vi "Sprinkler.vi"() -> ()   [LabVIEW 2020]
uses:
  Controls/ZoneSetupArray.ctl
  Controls/SprinklerStates.ctl
  <vilib>/Utility/file.llb/Read Delimited Spreadsheet (string).vi
panel:
  in  "Zone Setup Array":T1
  out "Controller Status":string
  out "Zone Indicators":T2
  in  "Water Pressure Sensor (%)":u32(slide) scale=0.0..100.0
  in  "Rain Sensor":bool
  in  "Run Selector":bool
  in  "Setup":bool
  in  "Start":bool
  in  "stop":bool
  # "Controls"
  # "Simulation Controls"
  # "Rain"
  # "No Rain"
  # "Continuous"
  # "Single"
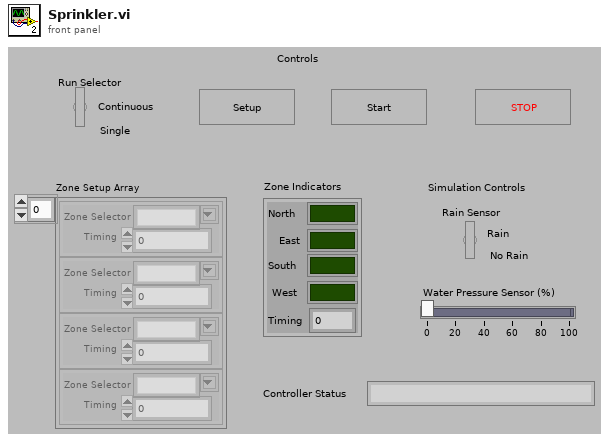
[diagram p1: front panel]
types:
  T1 = typedef "ZoneSetupArray.ctl" = cluster{"Zone Selector":string, "Timing":dbl}[]
  T2 = cluster{"North":bool, "East":bool, "South":bool, "West":bool, "Timing":u32}
  T3 = typedef "SprinklerStates.ctl" = cluster{enum16{"Default", "Init", "Setup", "Start", "Stop"}, variant}
  T4 = enum8{"Enabled", "Disabled", "Disabled and Grayed Out"}
  T5 = enum16{"Default", "Init", "Setup", "Start", "Stop"}
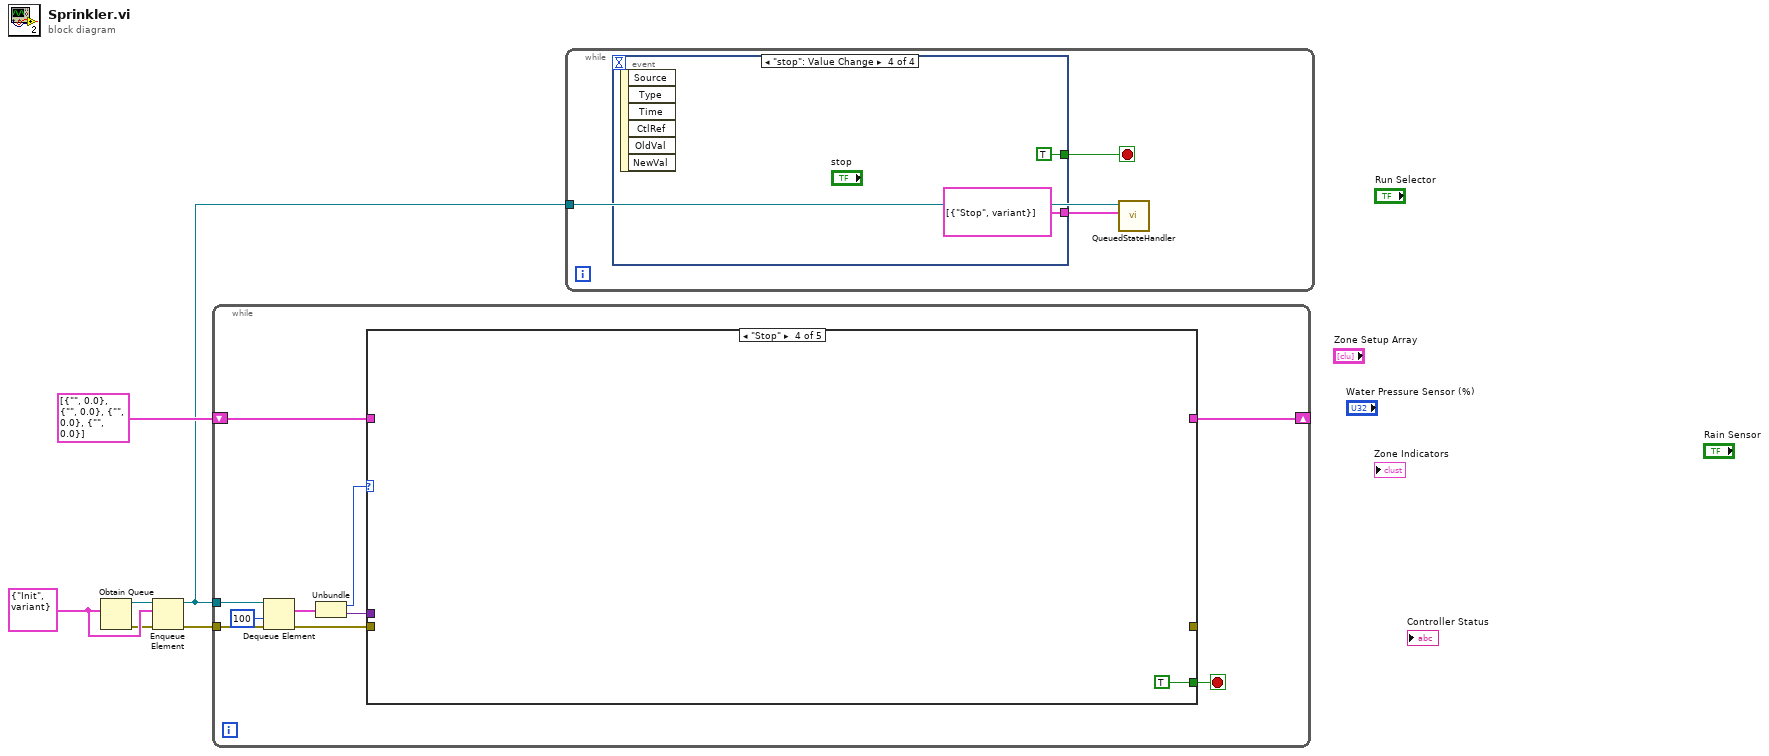
[diagram p0: block diagram]
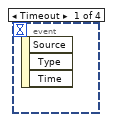
[diagram p2: hidden frame]
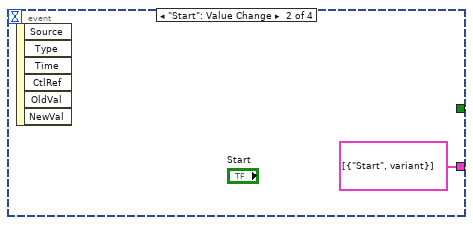
[diagram p3: hidden frame]
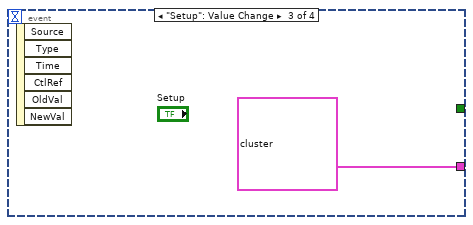
[diagram p4: hidden frame]
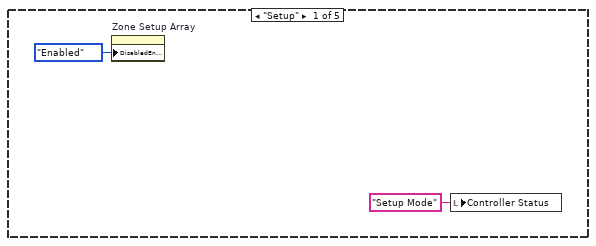
[diagram p5: hidden frame]
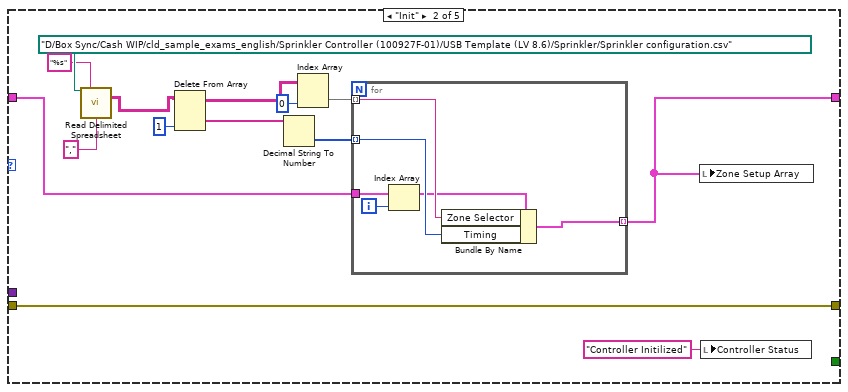
[diagram p6: hidden frame]
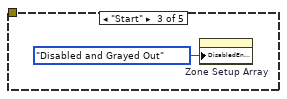
[diagram p7: hidden frame]
diagram:
  w5 = T3 {enum."Init", variant}
  n1 = Obtain Queue(element data type=w5) -> (queue out=w6:refnum<queue>, error out=w4:errorcluster)  [unwired: 4 in, 1 out]
  n2 = Enqueue Element(queue=w6, element=w5, error in (no error)=w4) -> (queue out=w1:refnum<queue>, error out=w3:errorcluster)  [unwired: 1 in, 1 out]
  n3 = while {
    tunnel: w1 -> [w16]
    tunnel: w3 -> [w15]
    shift-right: [w9] -> _
    shift-left: T1 [{"Zone Selector"="", "Timing"=0.0}, {"Zone Selector"="", "Timing"=0.0}, {"Zone Selector"="", "Timing"=0.0}, {"Zone Selector"="", "Timing"=0.0}] ("Zone Setup Array") -> [w10]
    stop <- w7 stop-if-true
    n4 = Dequeue Element(queue=w16, timeout in ms (-1)=100, error in (no error)=w15) -> (element=w13:T3, error out=w8:errorcluster)  [unwired: 2 out]
    n5 = Unbundle(w13) -> (w12:T5, w11:variant)
    n6 = case shown="\"Stop\"" w12 {
      tunnel: w11 -> [_ _ _ _ _]
      tunnel: w10 -> [_ w22 _ _ _]
      tunnel: [_ w20 _ _ _] -> w9
      tunnel: w8 -> [_ w21 _ _ _]
      tunnel: [_ w21 _ _ _] -> _
      tunnel: [_ _ _ TRUE _] -> w7
      frame "Setup" {
        n7 = property on="Zone Setup Array" class="Arr (strict)"("DisabledEnum"=T4."Enabled" ("Disabled")) -> ()  [unwired: 2 in, 2 out]
        n8 = local write "Controller Status"("Setup Mode" ("Controller Status")) -> ()
      }
      frame "Init" {
        n9 = call-poly <vilib>:"Read Delimited Spreadsheet.vi"("file path (dialog if empty)"=path "D:/Box Sync/Cash WIP/cld_sample_exams_english/Sprinkler Controller (100927F-01)/USB Template (LV 8.6)/Sprinkler/Sprinkler configuration.csv", "format (%s)"="%s" ("format (%d)"), "delimiter (\\t)"="," ("delimiter (\\t)")) -> ("all rows"=w27:string[][])  [unwired: 7 in, 5 out]
        n10 = Delete From Array(array=w27, index (col)=1 ("disabled index (col)")) -> (deleted portion=w29:string[], array with subset deleted=w25:string[][])  [unwired: 2 in]
        n11 = Decimal String To Number(string=w29) -> (number=w26:i32[])  [unwired: 2 in, 1 out]
        n12 = Index Array(array=w25, index (col)=0 ("disabled index (col)")) -> (element=w24:string[])  [unwired: 1 in]
        n13 = for {
          tunnel: w22 -> [w37]
          tunnel: [w38] -> w20 mode=indexing
          tunnel: w26 -> [w36] mode=indexing
          tunnel: w24 -> [w35] mode=indexing
          i -> [w33]
          n14 = Index Array(array=w37, index=w33) -> (element=w34:cluster{"Zone Selector":string, "Timing":dbl})
          n15 = Bundle By Name(cluster=w34, "Zone Selector"=w35, "Timing"=w36) -> (w38:cluster{"Zone Selector":string, "Timing":dbl})
        }
        n16 = local write "Zone Setup Array"(w20) -> ()
        n17 = local write "Controller Status"("Controller Initilized" ("Controller Status")) -> ()
      }
      frame "Start" {
        n18 = property on="Zone Setup Array" class="Arr (strict)"("DisabledEnum"=T4."Disabled and Grayed Out" ("Disabled")) -> ()  [unwired: 2 in, 2 out]
      }
      frame "Stop" {
      }
      frame "Default" {
      }
    }
  }
  n19 = while {
    tunnel: w1 -> [w42]
    stop <- w41 stop-if-true
    n20 = event shown="[3] \"stop\": Value Change" {
      selector: _ -> [_ _ _ _]
      dyn-events: _ -> [_ _ _ _]
      timeout: _ -> [_ _ _ _]
      tunnel: [_ T3[] [{enum."Start", variant}] T3[] [{enum."Stop", variant}, {enum."Setup", variant}] T3[] [{enum."Stop", variant}]] -> w43
      tunnel: [_ _ _ TRUE] -> w41
      event Timeout {
        n21 = event-data() -> ()  [unwired: 1 in, 3 out]
      }
      event "Start": Value Change {
        n22 = event-data() -> ()  [unwired: 1 in, 6 out]
      }
      event "Setup": Value Change {
        n23 = event-data() -> ()  [unwired: 1 in, 6 out]
      }
      event "stop": Value Change {
        n24 = event-data() -> ()  [unwired: 1 in, 6 out]
      }
    }
    n25 = call "QueuedStateHandler.vi"("Array"=w43, "queue out"=w42) -> ()  [unwired: 9 in, 1 out]
  }
